vi "Get Moving Status.vi"(8 "error in (no error)":errorcluster, 11 "SIM Motion Controller in":refnum<class "Fine SIM Motion Controller.lvclass">) -> (0 "error out":errorcluster, 2 "Moving?":bool, 3 "SIM Motion Controller out":refnum<class "Fine SIM Motion Controller.lvclass">)   [LabVIEW 2022 SP3, in "Fine SIM Motion Controller.lvclass"]
uses:
  Fine SIM Motion Controller.lvclass
  Fine SIM Motion Controller.lvclass/Fine SIM Motion Controller.ctl
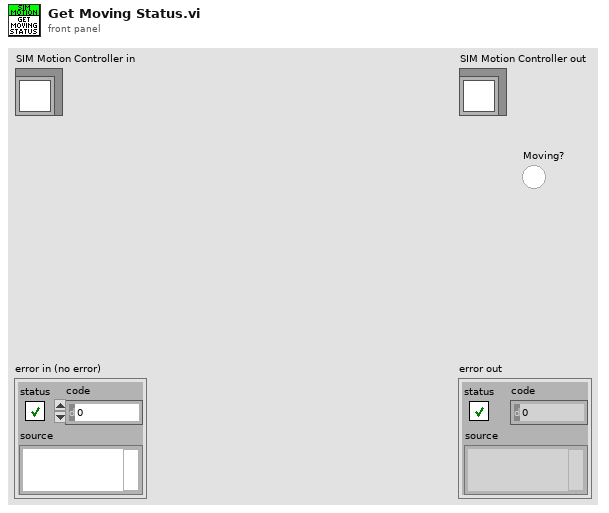
[diagram p1: front panel]
types:
  T1 = typedef "Parent SIM Motion Controller.lvclass/Axis Data.ctl" = cluster{"Axis Parameters":T2, "Axis Settings":T3, "Time Stamp":timestamp}
  T2 = typedef "Parent SIM Motion Controller.lvclass/Axis Parameters.ctl" = cluster{"Moving":bool, "Homed":bool, "Desired Position":dbl, "Current Positon":dbl, "Current Speed":dbl}
  T3 = typedef "Parent SIM Motion Controller.lvclass/Axis Settings.ctl" = cluster{"Speed":dbl, "Acceleration":dbl}
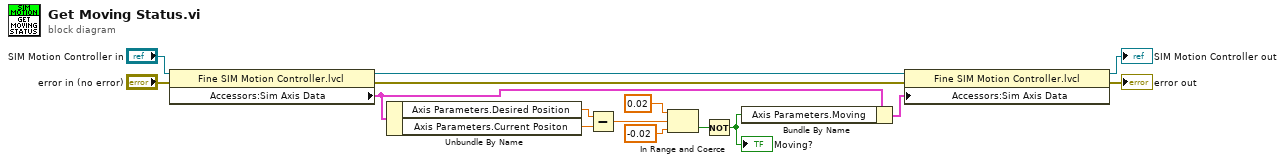
[diagram p0: block diagram]
diagram:
  n1 = property class="Fine SIM Motion Controller.lvcl"(reference="SIM Motion Controller in", error in="error in (no error)") -> (reference out=w13:refnum<class "Fine SIM Motion Controller.lvclass">, error out=w11:errorcluster, "Accessors:Sim Axis Data"=w2:T1)
  n2 = Unbundle By Name(w2) -> ("Axis Parameters.Desired Position"=w8:dbl, "Axis Parameters.Current Positon"=w7:dbl)
  n3 = Subtract(x=w8, y=w7) -> (x-y=w6:dbl)
  n4 = In Range and Coerce(upper limit=0.02, x=w6, lower limit=-0.02) -> (In Range?=w3:bool)  [unwired: 1 out]
  n5 = Not(x=w3) -> (.not. x?=w9:bool)
  "Moving?" <- w9
  n6 = Bundle By Name(cluster=w2, "Axis Parameters.Moving"=w9) -> (w1:T1)
  n7 = property class="Fine SIM Motion Controller.lvcl"(reference=w13, error in=w11, "Accessors:Sim Axis Data"=w1) -> (reference out=→"SIM Motion Controller out":refnum<class "Fine SIM Motion Controller.lvclass">, error out=→"error out":errorcluster)
